vi "Set Waveform Shape.vi"(8 "error in (no error)":errorcluster, 9 "Waveform Shape":T1 items=["Sinusoid", "Square", "Pulse", "Ramp", "PRNoise", "DC", "SINC", "Gaussian", "Lorentz", "ERise", "EDecay", "Haversine", "User 1", "User 2", "User 3", "User 4", "EMemory", "EFile"], 10 "Channel (0: Channel 1)":T2 items=["Channel 1", "Channel 2"], 11 "VISA resource name":refnum<visa-resource-name>) -> (0 "error out":errorcluster, 3 "VISA resource name out":refnum<visa-resource-name>)   [LabVIEW 2012, in "Tektronix AFG 3000 Series.lvlib"]
doc: "Sets the shape of the output waveform on a Tektronix AFG 3000 series function generator. <B>Notes:</B> if the waveform you select is not compatible with the current run mode, it will automatically change to continuous. Also, changing the output waveform may change the frequency, since the range of allowed frequencies will be different."
uses:
  Tektronix AFG 3000 Series.lvlib
  controls.llb/Channel.ctl
  controls.llb/Waveform Shape.ctl
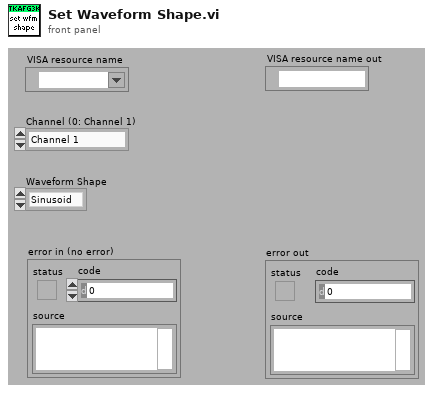
[diagram p1: front panel]
types:
  T1 = typedef "Waveform Shape.ctl" = u16
  T2 = typedef "Channel.ctl" = u16
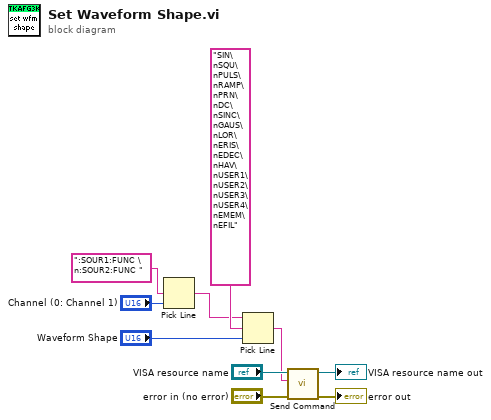
[diagram p0: block diagram]
diagram:
  n1 = Pick Line(multi-line string=":SOUR1:FUNC \n:SOUR2:FUNC ", line index="Channel (0: Channel 1)") -> (output string=w4:string)  [unwired: 1 out]
  n2 = Pick Line(string ("")=w4, multi-line string="SIN\nSQU\nPULS\nRAMP\nPRN\nDC\nSINC\nGAUS\nLOR\nERIS\nEDEC\nHAV\nUSER1\nUSER2\nUSER3\nUSER4\nEMEM\nEFIL", line index="Waveform Shape") -> (output string=w2:string)
  n3 = call "Send Command.vi"("error in (no error)"="error in (no error)", "write buffer"=w2, "VISA resource name"="VISA resource name") -> ("error out"=→"error out":errorcluster, "VISA resource name out"=→"VISA resource name out":refnum<visa-resource-name>)  [unwired: 7 out]
